vi "Blink.vi"   [LabVIEW 2012]
types:
  T1 = typedef "BotSpeak_Control.ctl" = cluster{"Address":string, "Reply EOF":string, "Hardware":string, "Retries":i8, "Timeout":i32}
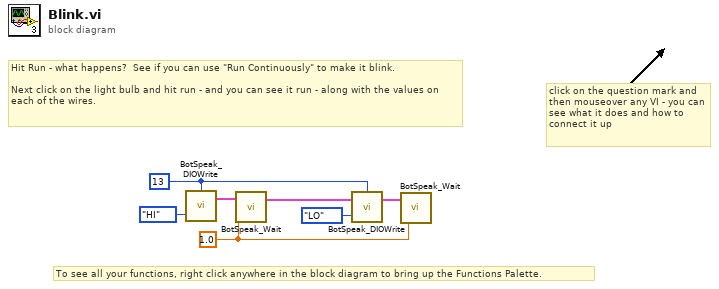
[diagram p0: block diagram]
diagram:
  w1 = 1.0 ("Wait (sec)")
  w5 = u32 13 ("DIO Line")
  # "To see all your functions, right click anywhere in the block diagram to bring up the Functions Palette."
  # "click on the question mark and then mouseover any VI - you can see what it does and how to connect it up"
  # "Hit Run - what happens?  See if you can use \"Run Continuously\" to make it blink.\n\nNext click on the light bulb and hit run - and you can see it run - along with the values on each of the wires."
  n1 = call <userlib>:"BotSpeak_DIOWrite.vi"("State"=enum32{"LO", "HI"}."HI", "DIO Line"=w5) -> ("Bot Settings"=w4:T1)  [unwired: 1 in, 1 out]
  n2 = call <userlib>:"BotSpeak_Wait.vi"("Wait (sec)"=w1, "Bot Settings"=w4) -> ("Bot Settings"=w3:T1)  [unwired: 1 in]
  n3 = call <userlib>:"BotSpeak_DIOWrite.vi"("State"=enum32{"LO", "HI"}."LO", "Bot Settings"=w3, "DIO Line"=w5) -> ("Bot Settings"=w2:T1)  [unwired: 1 out]
  n4 = call <userlib>:"BotSpeak_Wait.vi"("Wait (sec)"=w1, "Bot Settings"=w2) -> ()  [unwired: 1 in, 1 out]
